vi "TCU_CmdStr.vi"(1 "TCU":T1 {"仪表显示档位状态" items=["无显示", "显示P", "显示R", "显示N", "显示D", "显示M1", "显示M2", "显示M3", "显示M4", "显示M5", "显示M6", "显示M7", "显示M1+", "显示M2+", "显示M3+", "显示M4+", "显示M5+", "显示M6+", "显示M2-", "显示M3-", "显示M4-", "显示M5-", "显示M6-", "显示M7-", "无效", "预留"]; "TCU档位模式" items=["未定义", "P", "R", "N", "D", "M", "预留", "无效"]}) -> (0 "CmdStr":string)   [LabVIEW 2013]
uses:
  TCU_113.ctl
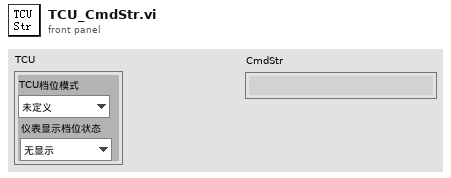
[diagram p1: front panel]
types:
  T1 = typedef "TCU_113.ctl" = cluster{"TCU档位模式":u8, "仪表显示档位状态":u8}
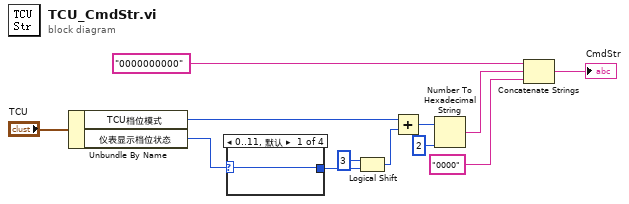
[diagram p0: block diagram]
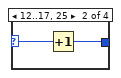
[diagram p2: hidden frame]
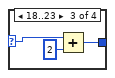
[diagram p3: hidden frame]
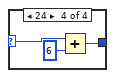
[diagram p4: hidden frame]
diagram:
  n1 = Unbundle By Name("TCU") -> ("TCU档位模式"=w2:u8, "仪表显示档位状态"=w1:u8)
  n2 = case shown="0..11, 默认" w1 {
    selector: w1 -> [w13 w15 w17 w20]
    tunnel: [w13 w14 w18 w21] -> w12
    frame 0..11, Default {
    }
    frame 12..17, 25 {
      n3 = Increment(x=w15) -> (x+1=w14:u8)
    }
    frame 18..23 {
      n4 = Add(x=w17, y=u8 2) -> (x+y=w18:u8)
    }
    frame 24 {
      n5 = Add(x=w20, y=u8 6) -> (x+y=w21:u8)
    }
  }
  n6 = Logical Shift(y=u8 3, x=w12) -> (x << y=w10:u8)
  n7 = Add(x=w2, y=w10) -> (x+y=w9:u8)
  n8 = Number To Hexadecimal String(1:i16 2 ("宽度(-)"), 2:w9) -> (0:w6:string)
  n9 = Concatenate Strings("0000000000", w6, "0000") -> (→"CmdStr":string)
